vi "6_物体识别.vi"() -> ()   [LabVIEW 2020]
panel:
  in  "Use File Path Image Type":bool=TRUE
  in  "停止":bool
  out "Image 2":T1(plugin-control)
  out "error out":errorcluster
  out "物体数量":i32
  in  "Settings":T2={"Objects"=0, "Threshold"=128, "Reject Border"=FALSE, "Fill Holes"=FALSE, "Min Object Size"=FALSE, "Min Size"=3, "Max Object Size"=FALSE, "Max Size"=100, "Show Search Area"=FALSE, "Show Center"=TRUE, "Show Bounding Box"=TRUE} {"Objects" items=["Bright Objects", "Dark Objects"]; "Threshold" min=1 max=999999999 step=1; "Max Size" min=1 max=999999999 step=1; "Min Size" min=1 max=999999999 step=1}
  out "Image":T1(plugin-control)
  in  "要检测的文件路径":path
  in  "Image Type":T3 items=["Grayscale (U8)", "Grayscale (I16)", "Grayscale (SGL)", "Complex (CSG)", "RGB (U32)", "HSL (U32)", "RGB (U64)", "Grayscale (U16)"]
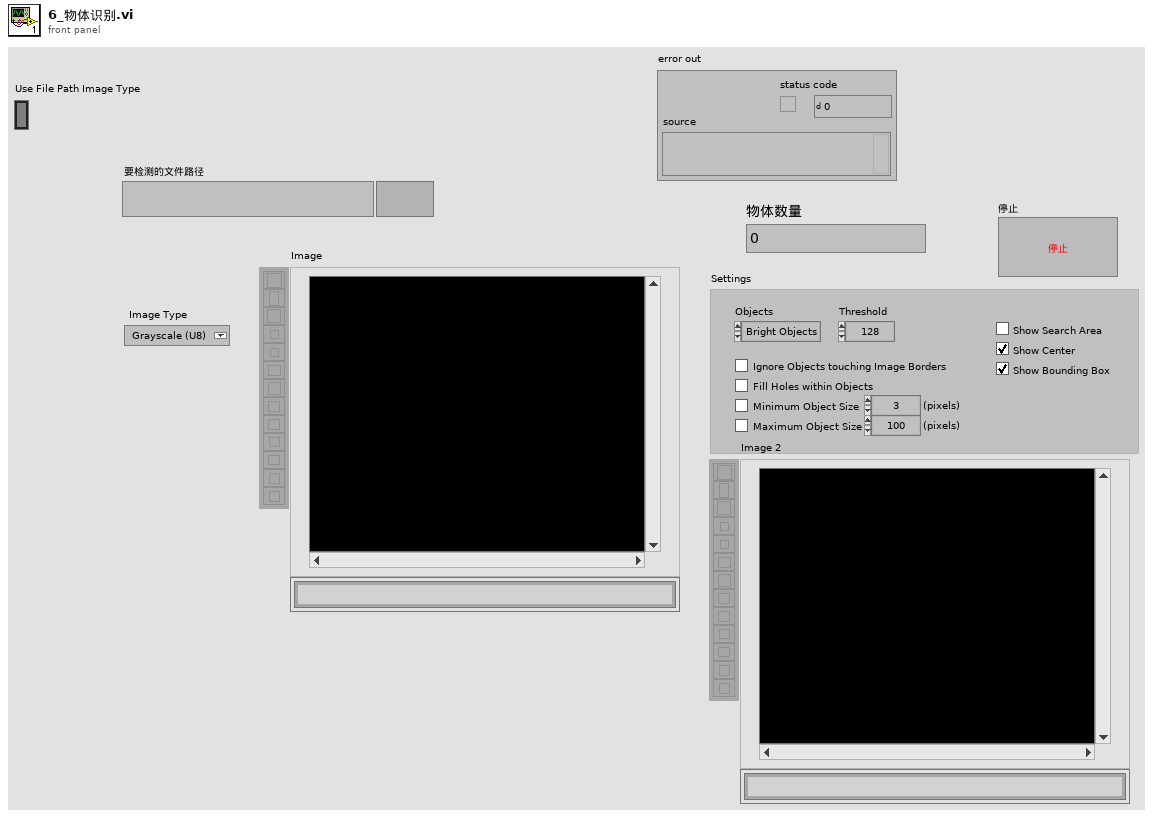
[diagram p1: front panel]
types:
  T1 = typedef "IMAQ Image.ctl" = refnum<image>
  T2 = cluster{"Objects":u16, "Threshold":i32, "Reject Border":bool, "Fill Holes":bool, "Min Object Size":bool, "Min Size":i32, "Max Object Size":bool, "Max Size":i32, "Show Search Area":bool, "Show Center":bool, "Show Bounding Box":bool}
  T3 = typedef "Image Type" = u32
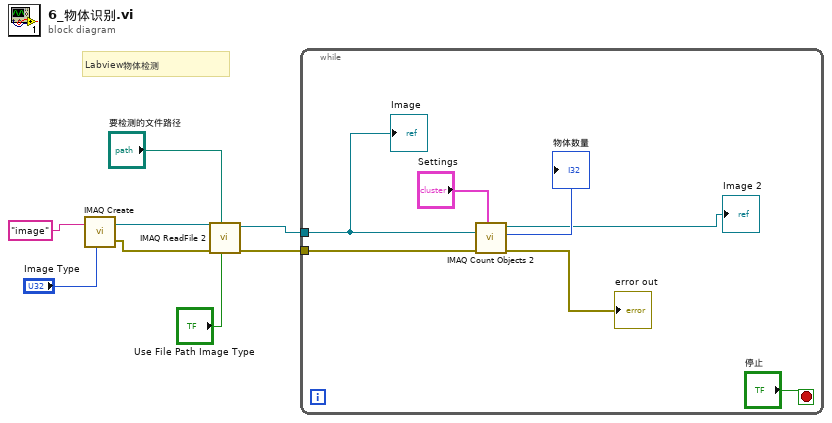
[diagram p0: block diagram]
diagram:
  # "Labview物体检测"
  n1 = call "IMAQ Create"("Image Name"="image", "Image Type"="Image Type") -> ("New Image"=w8:T1, "error out"=w3:errorcluster)  [unwired: 3 in]
  n2 = call "IMAQ ReadFile 2"("Use File Path Image Type"="Use File Path Image Type", "File Path"="要检测的文件路径", "error in (no error)"=w3, "Image"=w8) -> ("error out"=w2:errorcluster, "Image Out"=w4:T1)  [unwired: 3 in, 3 out]
  n3 = while {
    tunnel: w4 -> [w15]
    tunnel: w2 -> [w12]
    stop <- "停止" stop-if-true
    n4 = call "IMAQ Count Objects 2"("Settings"="Settings", "error in (no error)"=w12, "Image"=w15) -> ("error out"=→"error out":errorcluster, "Number of Objects"=→"物体数量":i32, "Image Out"=→"Image 2":T1)  [unwired: 4 in, 2 out]
    "Image" <- w15
  }
